vi "Lutron Query.vi"(8 "error in (no error)":errorcluster, 11 "VISA resource name in":refnum<visa-resource-name>) -> (0 "error out":errorcluster, 1 "All Found":string[](array[string]), 2 "First out":string, 3 "VISA resource name out":refnum<visa-resource-name>)   [LabVIEW 2016, in "Lutron QS Control Protocol.lvlib" / "Lutron QS Object.lvclass"]
uses:
  Lutron QS Object.lvclass
panel:
  out "return count 2":u32
  out "read buffer 3":string
  out "Current length":i32
  out "i":i32
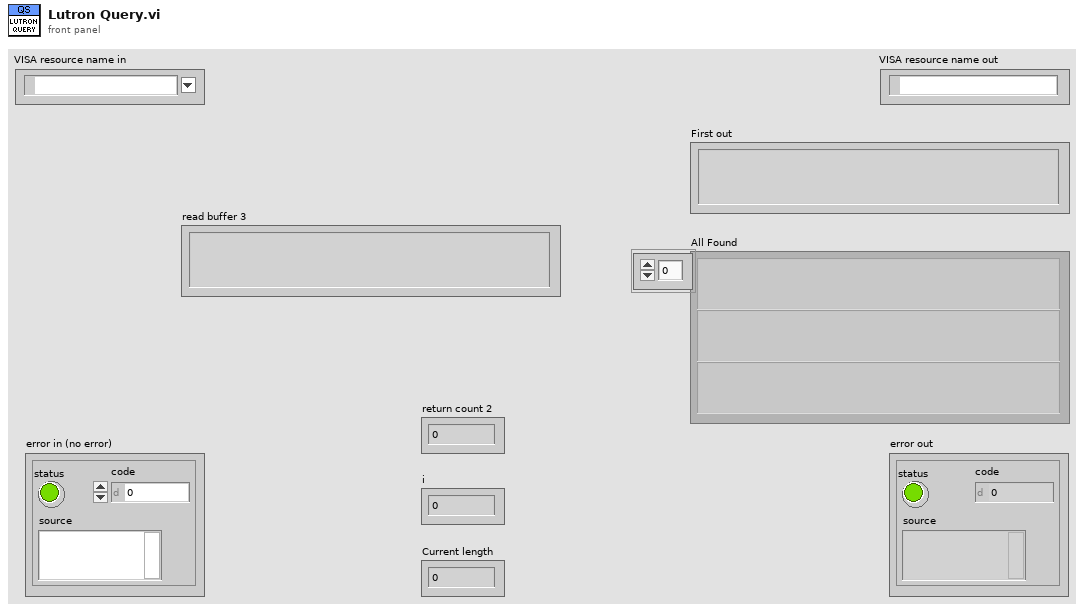
[diagram p1: front panel]
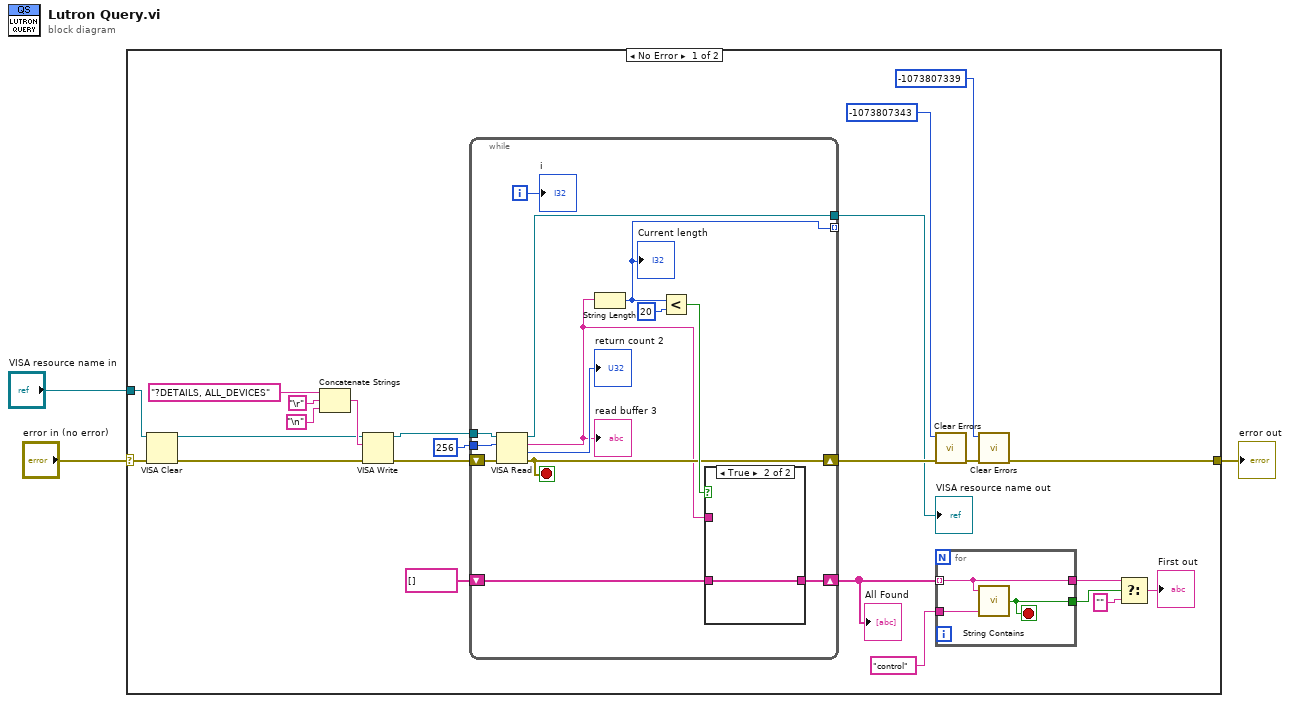
[diagram p0: block diagram]
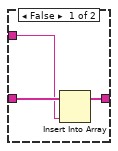
[diagram p2: hidden frame]
diagram:
  n1 = case shown="No Error" "error in (no error)" {
    selector: "error in (no error)" -> [w27 w48]
    tunnel: [w7 w48] -> w2
    tunnel: "VISA resource name in" -> [w26 _]
    frame No Error {
      n2 = VISA Clear(VISA resource name=w26, error in (no error)=w27) -> (VISA resource name out=w20:refnum<visa-resource-name>, error out=w19:errorcluster)
      n3 = Concatenate Strings("?DETAILS, ALL_DEVICES" ("string"), "\r", "\n") -> (w25:string)
      n4 = VISA Write(VISA resource name=w20, write buffer=w25, error in (no error)=w19) -> (VISA resource name out=w17:refnum<visa-resource-name>, error out=w16:errorcluster)  [unwired: 1 out]
      n5 = while {
        tunnel: w17 -> [w43]
        shift-right: [w33] -> w11
        shift-left: w16 -> [w42]
        tunnel: u32 256 ("byte count") -> [w39]
        shift-right: [w37] -> w5
        shift-left: string[] [] -> [w38]
        tunnel: [w36] -> _ mode=indexing
        tunnel: [w31] -> w4
        i -> [w40]
        stop <- w33 stop-if-true
        n6 = VISA Read(VISA resource name=w43, byte count=w39, error in (no error)=w42) -> (VISA resource name out=w31:refnum<visa-resource-name>, read buffer=w32:string, return count=→"return count 2":u32, error out=w33:errorcluster)
        "read buffer 3" <- w32
        n7 = String Length(string=w32) -> (length=w36:i32)
        "Current length" <- w36
        n8 = Less?(x=w36, y=20) -> (x < y?=w34:bool)
        n9 = case shown="True" w34 {
          tunnel: w38 -> [w46 w47]
          tunnel: w32 -> [w45 _]
          tunnel: [w44 w47] -> w37
          frame False {
            n10 = Insert Into Array(array=w46, new element=w45) -> (w44:string[])  [unwired: 1 in]
          }
          frame True {
          }
        }
        "i" <- w40
      }
      "All Found" <- w5
      "VISA resource name out" <- w4
      n11 = call <vilib>:"Clear Errors.vi"("error in (no error)"=w11, "specific error code to clear (0: all)"=-1073807343 ("code")) -> ("error out"=w8:errorcluster)  [unwired: 4 in, 1 out]
      n12 = for {
        tunnel: "control" -> [w30]
        tunnel: w5 -> [w28] mode=indexing
        tunnel: [w29] -> w15
        tunnel: [w28] -> w14
        stop <- w29 stop-if-true
        n13 = call "String Contains.vi"("Regular expression"=w30, "Input String"=w28) -> ("Found?"=w29:bool)  [unwired: 2 in, 1 out]
      }
      n14 = call <vilib>:"Clear Errors.vi"("error in (no error)"=w8, "specific error code to clear (0: all)"=-1073807339 ("code")) -> ("error out"=w7:errorcluster)  [unwired: 4 in, 1 out]
      n15 = Select(t=w14, s=w15, f="") -> (s? t:f=→"First out":string)
    }
    frame Error {
    }
  }
  "error out" <- w2
